vi "zlgcan_demo_USBCANFD.vi"() -> ()   [LabVIEW 2018]
uses:
  data_type/ZCAN_InitCAN_setting_USBCANFD.ctl
panel:
  in  "是否使用电阻":u8(ring) items=["不使用终端电阻", "使用终端电阻"]
  in  "数据域波特率":u32(ring)=500000 items=["1Mbps"=1000000, "800kbps"=800000, "500kbps"=500000, "250kbps"=250000, "125kbps"=125000, "100kbps"=100000, "50kbps"=50000]
  in  "工作模式":u8(ring) items=["正常", "只听"]
  in  "自定义波特率字符输入":string
  in  "使用自定义波特率？":bool
  in  "仲裁域波特率":u32(ring)=500000 items=["1Mbps"=1000000, "800kbps"=800000, "500kbps"=500000, "250kbps"=250000, "125kbps"=125000, "100kbps"=100000, "50kbps"=50000]
  in  "通道索引":u32(ring) items=["0", "1", "2", "3"]
  in  "设备索引":u32(ring) items=["0", "1", "2", "3"]
  in  "设备类型":u32(ring)=41 items=["PCI-9810"=2, "USBCAN-II"=4, "USBCAN-E-U"=20, "PCIE-CANFD-100U"=38, "PCIE-CANFD-200U"=39, "PCIE-CANFD-400U"=40, "USBCANFD-200U"=41, "USBCANFD-100U"=42, "USBCANFD-MINI"=43, "云设备"=46]
  in  "开启CAN":bool
  in  "stop":bool
  in  "ID":u32 format="0x%08x"
  in  "数据长度(最大8字节)":u8=8 max=8
  in  "Data Byte 8":u8 caption="data88" format="%.0x"
  in  "Data Byte 7":u8 caption="data7" format="%.0x"
  in  "Data Byte 6":u8 caption="data6" format="%.0x"
  in  "Data Byte 5":u8 caption="data5" format="%.0x"
  in  "Data Byte 4":u8 caption="data4" format="%.0x"
  in  "Data Byte 3":u8 caption="data3" format="%.0x"
  in  "Data Byte 2":u8 caption="data2" format="%.0x"
  in  "Data Byte 1":u8 caption="data1" format="%.0x"
  in  "帧格式":u32(ring) items=["数据帧", "远程帧"]
  in  "发送方式":u32(ring) items=["正常发送", "单次发送", "自发自收", "单次自发自收"]
  in  "帧类型":u32(ring) items=["标准帧", "扩展帧"]
  in  "每次发送帧数":u32=1
  in  "发送":bool
  in  "ZCAN_InitCAN_Setting_USBCANFD":T1
  out "can_index_handle(out)":u32
  out "Device_handle(out)":u32
  out "已接收帧数":u32
  out "接收字符串显示":string caption="String"
  # "如果是使用CAN,\n两个波特率设置相同即可"
  # "停止程序前，需要先关闭CAN卡"
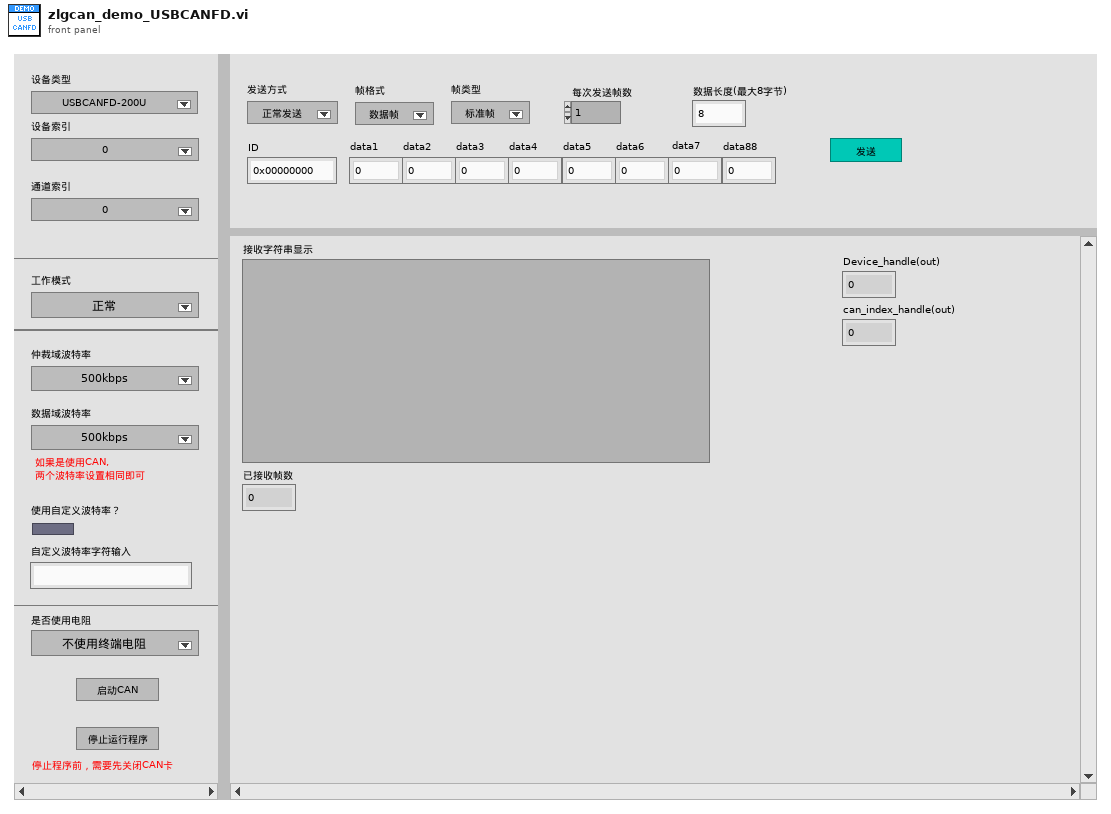
[diagram p1: front panel]
types:
  T1 = typedef "ZCAN_InitCAN_setting_USBCANFD.ctl" = cluster{"abitbaud":u32, "dbitbaud":u32, "baud_rate_custom？":bool, "RateCustom":string, "mode":u8}
  T2 = cluster{"[0]":u8, "[1]":u8, "[2]":u8, "[3]":u8, "[4]":u8, "[5]":u8, "[6]":u8, "[7]":u8}
  T3 = cluster{u32, u8, u8, u8, u8, cluster{"[0]":u8, "[1]":u8, "[2]":u8, "[3]":u8, "[4]":u8, "[5]":u8, "[6]":u8, "[7]":u8}, u64}[]
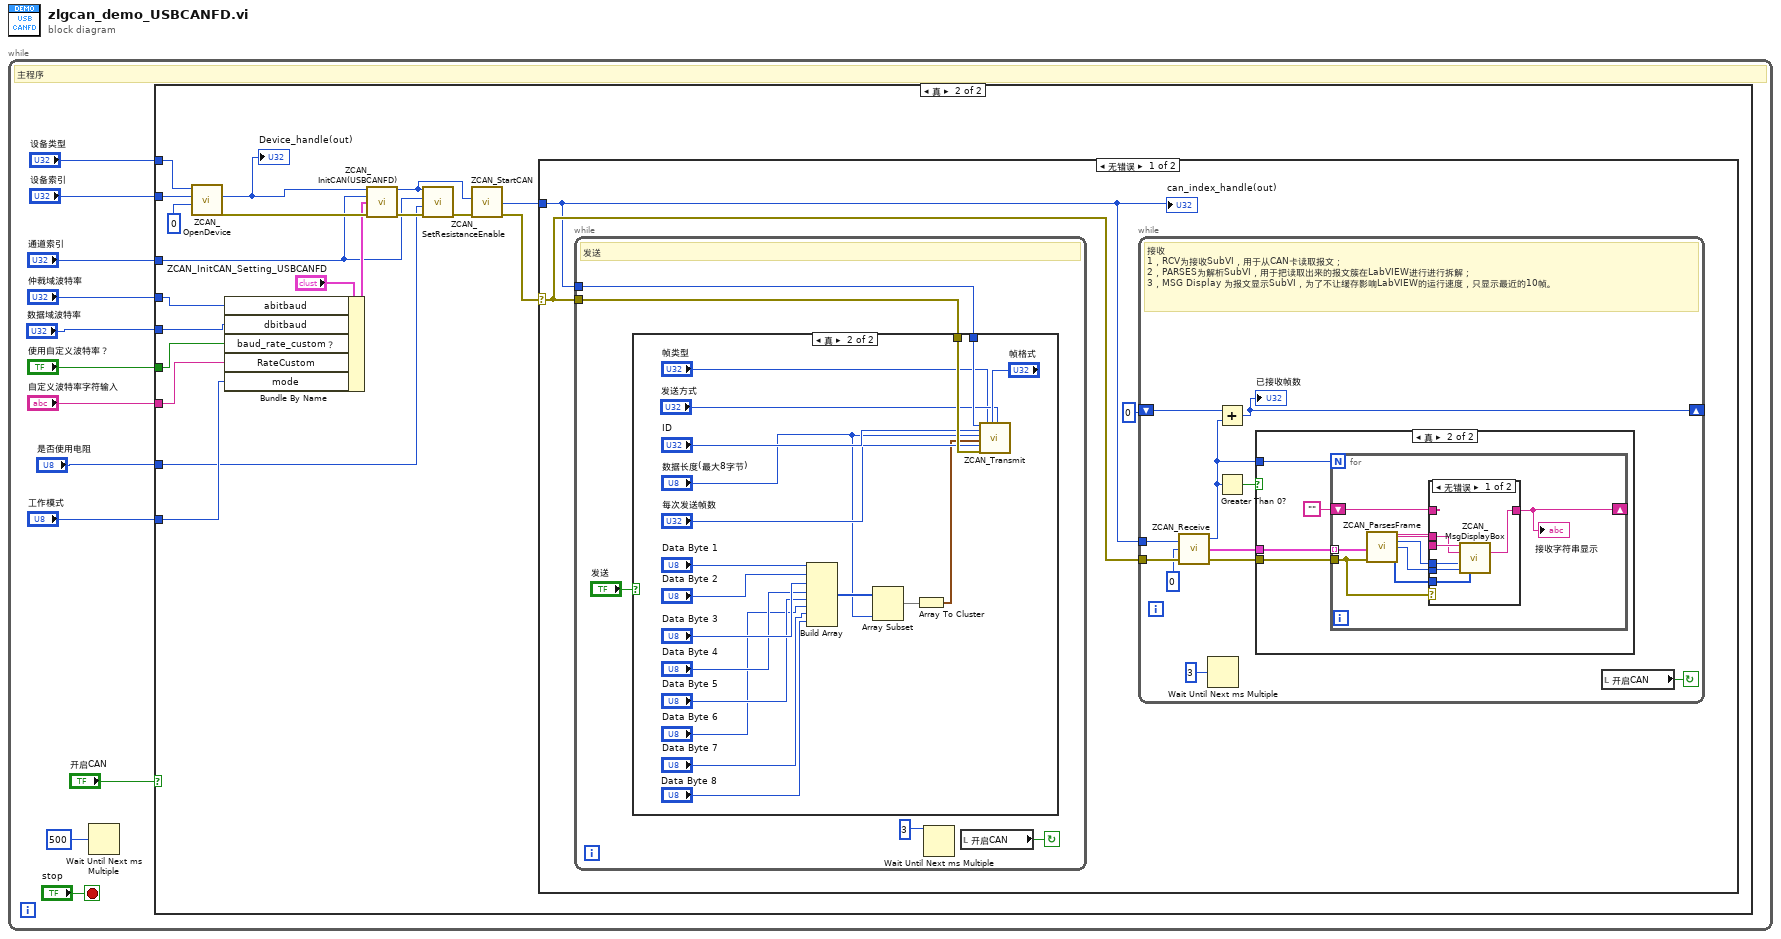
[diagram p0: block diagram]
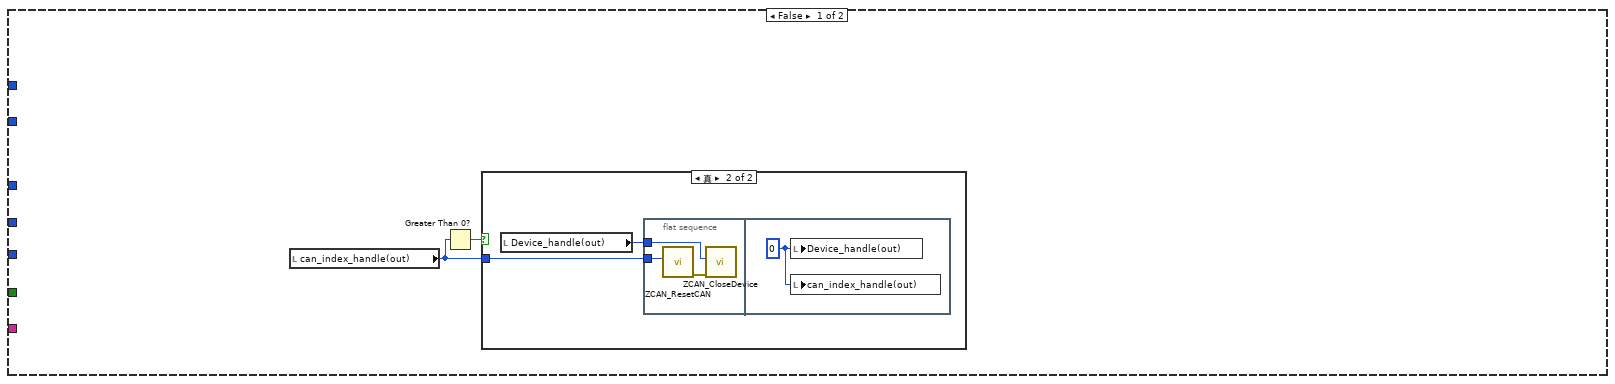
[diagram p2: hidden frame]
diagram:
  n1 = while {
    stop <- "stop" stop-if-true
    # "主程序"
    n2 = Wait Until Next ms Multiple(millisecond multiple=u32 500) -> ()  [unwired: 1 out]
    n3 = case shown="真" "开启CAN" {
      tunnel: "通道索引" -> [_ w23]
      tunnel: "仲裁域波特率" -> [_ w29]
      tunnel: "使用自定义波特率？" -> [_ w31]
      tunnel: "自定义波特率字符输入" -> [_ w28]
      tunnel: "工作模式" -> [_ w27]
      tunnel: "设备类型" -> [_ w37]
      tunnel: "设备索引" -> [_ w38]
      tunnel: "数据域波特率" -> [_ w30]
      tunnel: "是否使用电阻" -> [_ w22]
      frame False {
        # "关闭CAN卡"
        n4 = local read "can_index_handle(out)"() -> (w13:u32)
        n5 = Greater Than 0?(x=w13) -> (x > 0?=w14:bool)
        n6 = case shown="真" w14 {
          tunnel: w13 -> [_ w16]
          frame False {
          }
          frame True {
            n7 = local read "Device_handle(out)"() -> (w15:u32)
            n8 = flat-sequence {
              tunnel: w16 -> [w18]
              tunnel: w15 -> [w17]
              frame #0 {
                n9 = call "ZCAN_ResetCAN.vi"("can_handle"=w18) -> ("error out"=w19:errorcluster)  [unwired: 9 in, 1 out]
                n10 = call "ZCAN_CloseDevice.vi"("error in (no error)"=w19, "device_handle"=w17) -> ()  [unwired: 8 in, 2 out]
              }
              frame #1 {
                w20 = u32 0 ("can_index_handle(out)")
                n11 = local write "Device_handle(out)"(w20) -> ()
                n12 = local write "can_index_handle(out)"(w20) -> ()
              }
            }
          }
        }
      }
      frame True {
        n13 = call "ZCAN_OpenDevice.vi"("reserved"=0, "device_index"=w38, "device_type"=w37) -> ("error out"=w34:errorcluster, "DEVICE_HANDLE"=w33:u32)  [unwired: 7 in]
        "Device_handle(out)" <- w33
        n14 = Bundle By Name(cluster="ZCAN_InitCAN_Setting_USBCANFD", "abitbaud"=w29, "dbitbaud"=w30, "baud_rate_custom？"=w31, "RateCustom"=w28, "mode"=w27) -> (w26:T1)
        n15 = call "ZCAN_InitCAN(USBCANFD).vi"("device_hande"=w33, "can_index"=w23, "ZCAN_InitCAN_Setting_USBCANFD"=w26, "error in (no error)"=w34) -> ("can_index_handle"=w21:u32, "error out"=w25:errorcluster)  [unwired: 10 in]
        n16 = call "ZCAN_SetResistanceEnable.vi"("error in (no error)"=w25, "enable"=w22, "can_index"=w23, "can_index_handle"=w21) -> ("error out"=w24:errorcluster)  [unwired: 7 in]
        n17 = call "ZCAN_StartCAN.vi"("error in (no error)"=w24, "can_index_handle"=w21) -> ("error out"=w35:errorcluster, "can_index_handle(out)"=w36:u32)  [unwired: 7 in, 1 out]
        n18 = case shown="无错误" w35 {
          selector: w35 -> [w41 _]
          tunnel: w36 -> [w40 _]
          frame No Error {
            n19 = while {
              tunnel: w40 -> [w76]
              tunnel: w41 -> [w74]
              stop <- w75 continue-if-true
              # "发送"
              n20 = case shown="真" "发送" {
                tunnel: w76 -> [_ w97]
                tunnel: w74 -> [_ w96]
                frame False {
                }
                frame True {
                  n21 = Build Array("Data Byte 1", "Data Byte 2", "Data Byte 3", "Data Byte 4", "Data Byte 5", "Data Byte 6", "Data Byte 7", "Data Byte 8") -> (w83:u8[])
                  n22 = Array Subset(array=w83, length="数据长度(最大8字节)") -> (w81:u8[])  [unwired: 1 in]
                  n23 = Array To Cluster(array=w81) -> (cluster=w80:T2)
                  n24 = call "ZCAN_Transmit.vi"("can_index_handle"=w97, "ID"="ID", "数据长度"="数据长度(最大8字节)", "DATA"=w80, "每次发送帧数"="每次发送帧数", "error in (no error)"=w96, "帧类型"="帧类型", "帧格式"="帧格式", "发送方式"="发送方式") -> ()  [unwired: 10 in, 1 out]
                }
              }
              n25 = Wait Until Next ms Multiple(millisecond multiple=u32 3) -> ()  [unwired: 1 out]
              n26 = local read "开启CAN"() -> (w75:bool)
            }
            n27 = while {
              tunnel: w41 -> [w50]
              tunnel: w40 -> [w48]
              shift-right: [w51] -> _
              shift-left: 0 -> [w52]
              stop <- w43 continue-if-true
              # "接收\n1，RCV为接收SubVI，用于从CAN卡读取报文；\n2，PARSES为解析SubVI，用于把读取出来的报文簇在LabVIEW进行进行拆解；\n3，MSG Display 为报文显示SubVI，为了不让缓存影响LabVIEW的运行速度，只显示最近的10帧。"
              n28 = call "ZCAN_Receive.vi"("error in (no error)"=w50, "type"=u8 0, "can_handle"=w48) -> ("error out"=w46:errorcluster, "Receive"=w47:T3, "Receive_Num"=w45:u32)
              n29 = Wait Until Next ms Multiple(millisecond multiple=u32 3) -> ()  [unwired: 1 out]
              n30 = Add(x=w52, y=w45) -> (x+y=w51:u32)
              "已接收帧数" <- w51
              n31 = Greater Than 0?(x=w45) -> (x > 0?=w44:bool)
              n32 = case shown="真" w44 {
                tunnel: w45 -> [_ w57]
                tunnel: w47 -> [_ w56]
                tunnel: w46 -> [_ w55]
                frame False {
                }
                frame True {
                  n33 = for {
                    N: w57 -> [_]
                    tunnel: w56 -> [w64] mode=indexing
                    tunnel: w55 -> [w63]
                    shift-right: [w66] -> _
                    shift-left: "" -> [w65]
                    n34 = call "ZCAN_ParsesFrame.vi"("ZCAN_Receive_Data"=w64, "error in (no error)"=w63) -> ("帧格式"=w58:string, "帧类型"=w59:string, "ID"=w60:u32, "data_len"=w62:u8, "data"=w61:u8[])  [unwired: 8 in, 1 out]
                    n35 = case shown="无错误" w63 {
                      tunnel: [w72 w73] -> w66
                      tunnel: w65 -> [_ w73]
                      tunnel: w62 -> [w71 _]
                      tunnel: w61 -> [w70 _]
                      tunnel: w60 -> [w69 _]
                      tunnel: w59 -> [w68 _]
                      tunnel: w58 -> [w67 _]
                      frame No Error {
                        n36 = call "ZCAN_MsgDisplayBox.vi"("帧类型"=w68, "ID"=w69, "帧格式"=w67, "Message Data"=w70, "data_len"=w71) -> ("Output String"=w72:string)  [unwired: 10 in]
                      }
                      frame Error {
                      }
                    }
                    "接收字符串显示" <- w66
                  }
                }
              }
              n37 = local read "开启CAN"() -> (w43:bool)
            }
            "can_index_handle(out)" <- w40
          }
          frame Error {
          }
        }
      }
    }
  }
